vi "gpib_build_visa_resource_name.vi"(7 "test mode":bool, 8 "error in (no error)":errorcluster, 10 "GPIB settings":T1) -> (0 "error out":errorcluster, 1 "VISA Resource name 2":refnum<visa-resource-name>, 3 "VISA Resource name 1":refnum<visa-resource-name>)   [LabVIEW 2015]
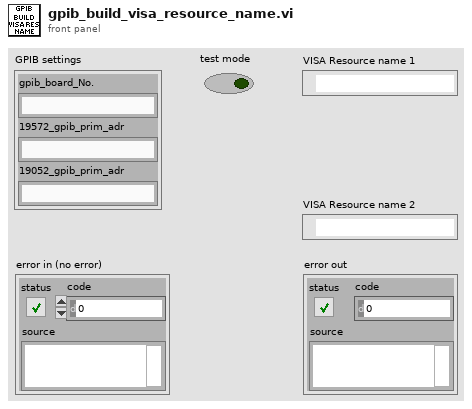
[diagram p1: front panel]
types:
  T1 = cluster{"gpib_board_No.":string, "19572_gpib_prim_adr":string, "19052_gpib_prim_adr":string}
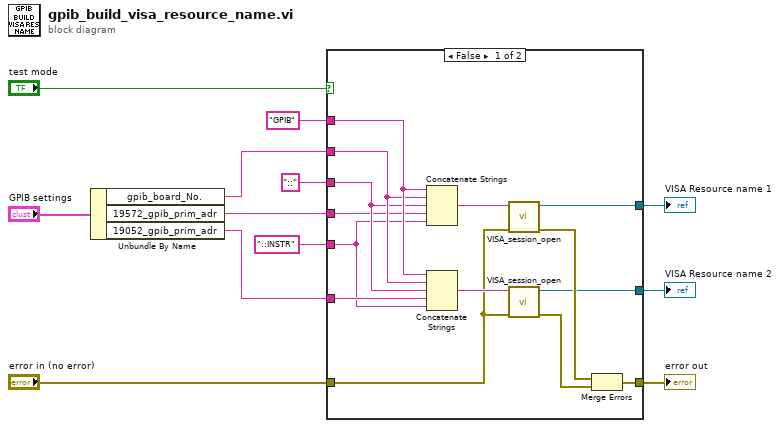
[diagram p0: block diagram]
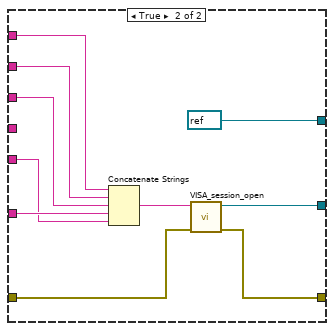
[diagram p2: hidden frame]
diagram:
  n1 = Unbundle By Name("GPIB settings") -> ("gpib_board_No."=w3:string, "19572_gpib_prim_adr"=w2:string, "19052_gpib_prim_adr"=w1:string)
  n2 = case shown="False" "test mode" {
    tunnel: w2 -> [w17 _]
    tunnel: w1 -> [w16 w28]
    tunnel: [w25 refnum<visa-resource-name> refnum ("VISA resource out 2")] -> w11
    tunnel: [w14 w29] -> w12
    tunnel: "error in (no error)" -> [w13 w35]
    tunnel: [w21 w34] -> w10
    tunnel: w3 -> [w19 w33]
    tunnel: "GPIB" -> [w20 w32]
    tunnel: "::" ("string") -> [w18 w31]
    tunnel: "::INSTR" -> [w15 w27]
    frame False {
      n3 = Concatenate Strings(w20, w19, w18, w17, w15) -> (w26:string)
      n4 = Concatenate Strings(w20, w19, w18, w16, w15) -> (w24:string)
      n5 = call "VISA_session_open.vi"("error in (no error)"=w13, "VISA resource name"=w26) -> ("error out"=w22:errorcluster, "VISA resource name out"=w25:refnum<visa-resource-name>)  [unwired: 8 in]
      n6 = call "VISA_session_open.vi"("error in (no error)"=w13, "VISA resource name"=w24) -> ("error out"=w23:errorcluster, "VISA resource name out"=w14:refnum<visa-resource-name>)  [unwired: 8 in]
      n7 = Merge Errors(w22, w23) -> (w21:errorcluster)
    }
    frame True {
      n8 = Concatenate Strings(w32, w33, w31, w28, w27) -> (w36:string)
      n9 = call "VISA_session_open.vi"("error in (no error)"=w35, "VISA resource name"=w36) -> ("error out"=w34:errorcluster, "VISA resource name out"=w29:refnum<visa-resource-name>)  [unwired: 8 in]
    }
  }
  "VISA Resource name 2" <- w12
  "VISA Resource name 1" <- w11
  "error out" <- w10
